vi "Create Configured.vi"(8 "error in (no error)":errorcluster, 10 "Report Interface":refnum<class "Report Interface.lvclass">) -> (0 "error out":errorcluster, 3 "Report Generator Out":refnum<class "Report Generator.lvclass">)   [LabVIEW 2020, in "Reports.lvlib" / "Report Generator.lvclass"]
uses:
  Report Generator.lvclass
  Report Interface/Report Interface.lvclass
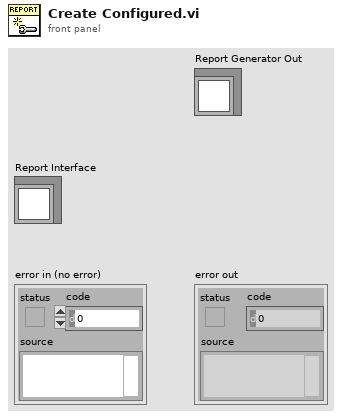
[diagram p1: front panel]
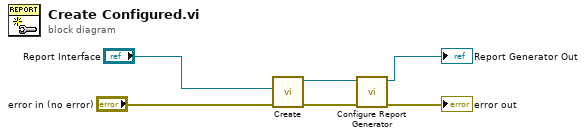
[diagram p0: block diagram]
diagram:
  n1 = call "Create.vi"("error in (no error)"="error in (no error)", "Report Interface"="Report Interface") -> ("error out"=w5:errorcluster, "Report Generator Out"=w3:refnum<class "Report Generator.lvclass">)  [unwired: 8 in]
  n2 = call "Configure Report Generator.vi"("error in (no error)"=w5, "Report Generator In"=w3) -> ("error out"=→"error out":errorcluster, "Report Generator Out"=→"Report Generator Out":refnum<class "Report Generator.lvclass">)  [unwired: 8 in]
